vi "ThermoV_ControlSweep_NoMean_RTDCalib_160817.vi"() -> ()   [LabVIEW 2013]
panel:
  out "subarray":dbl[](array[numeric])
  out "Array":dbl[](array[numeric])
  in  "Operate HVpp\nOutput Timer":bool caption="Reset"
  out "modular 13":dbl
  in  "Number of seconds for \neach HVpp case state":dbl=30.0
  out "Elapsed Time (s)":dbl
  out "DC Value":dbl[](array[numeric]) format="%#.6f"
  in  "Saving Avg?":bool
  in  "Filename":path=path "trial_1.lvm"
  in  "STOP":bool
  out "Peak2Peak V":dbl[](array[numeric])
  out "Waveform Chart":dynamicdata(graph)
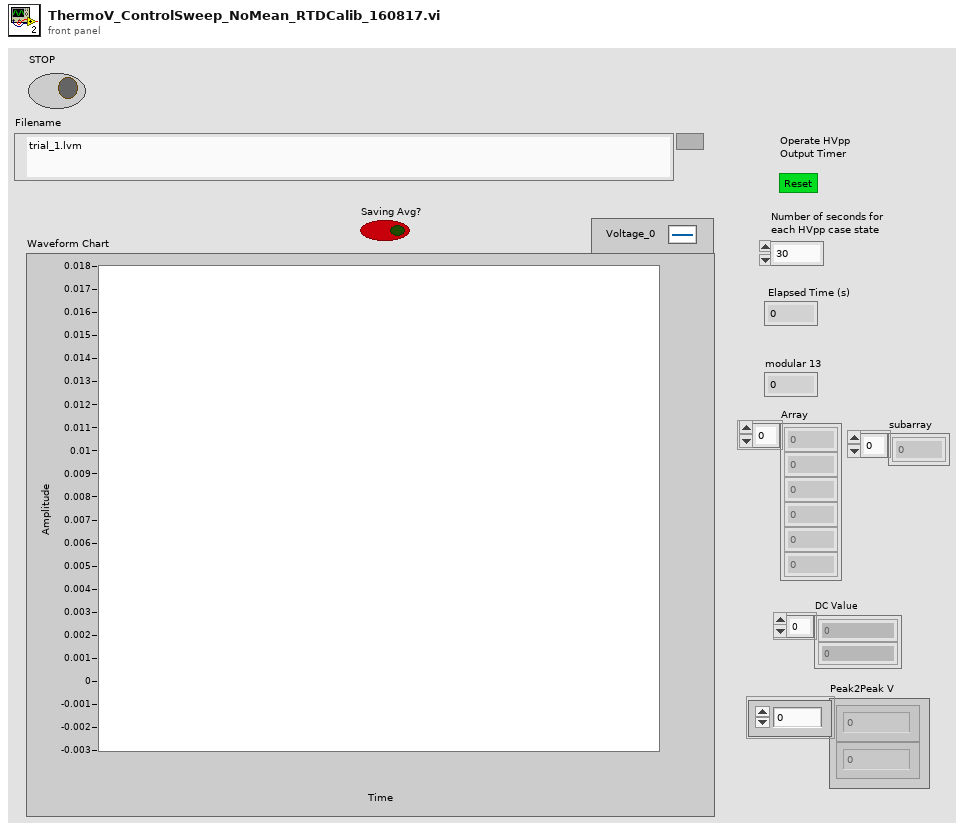
[diagram p1: front panel]
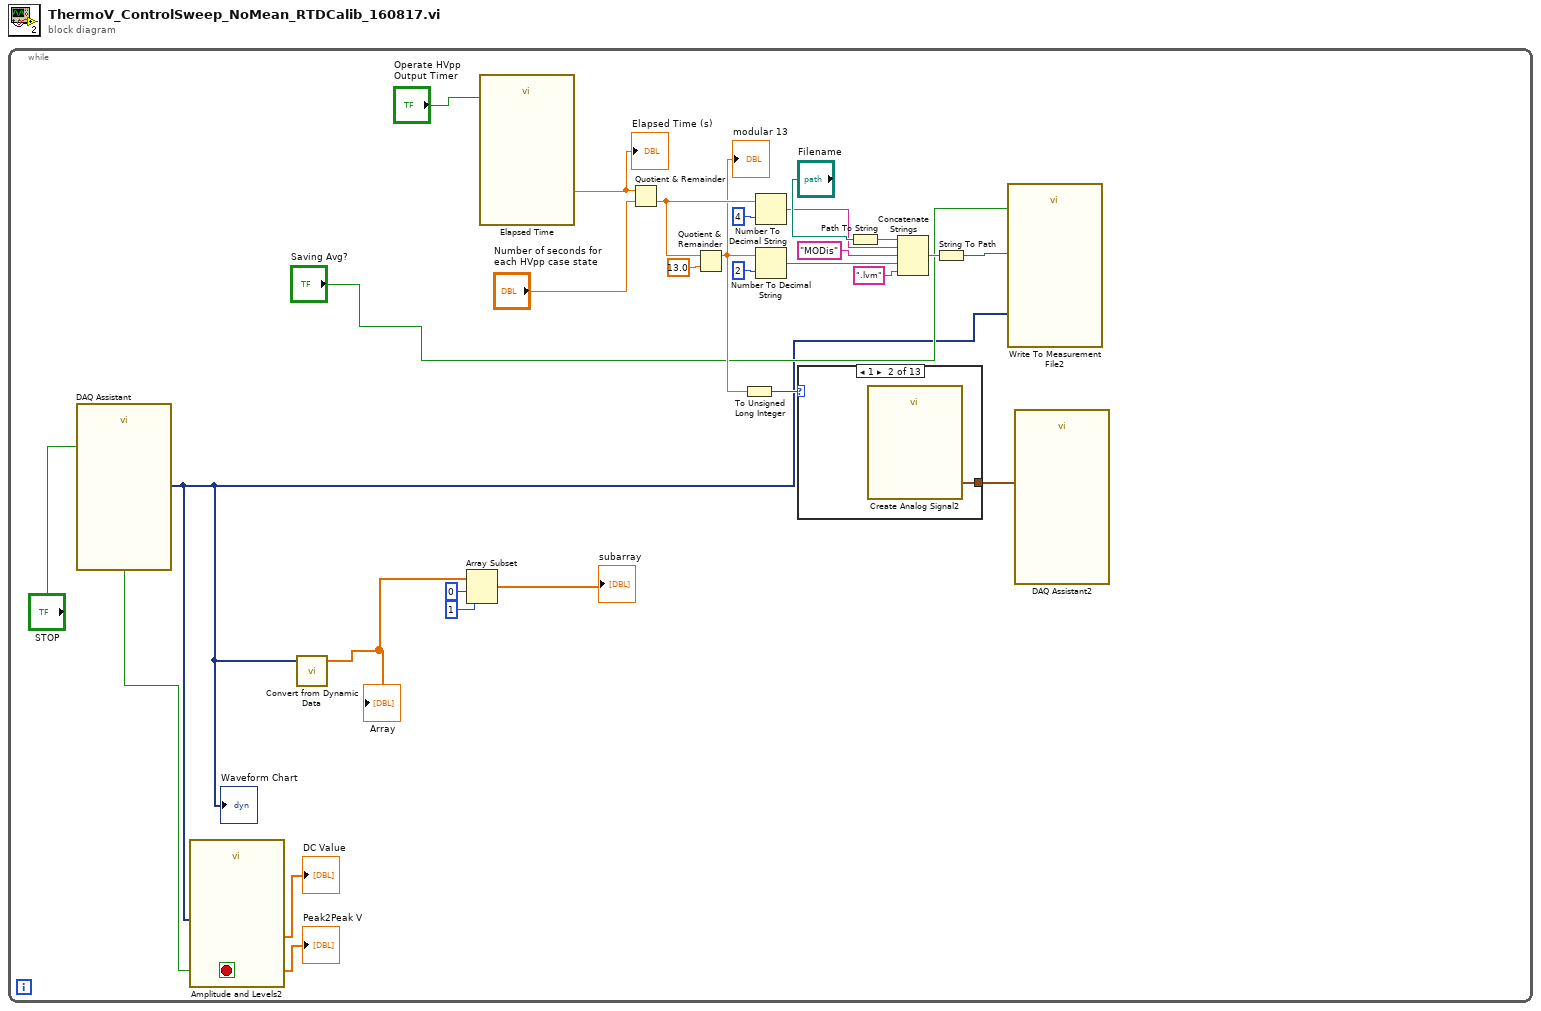
[diagram p0: block diagram]
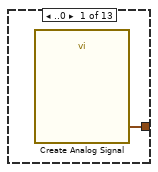
[diagram p2: hidden frame]
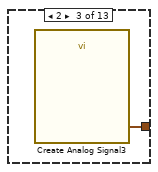
[diagram p3: hidden frame]
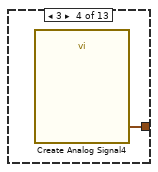
[diagram p4: hidden frame]
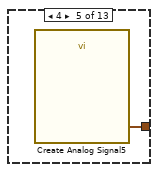
[diagram p5: hidden frame]
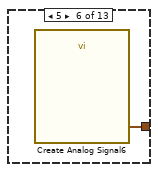
[diagram p6: hidden frame]
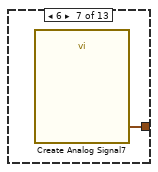
[diagram p7: hidden frame]
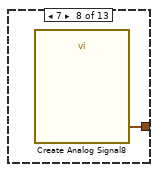
[diagram p8: hidden frame]
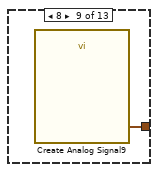
[diagram p9: hidden frame]
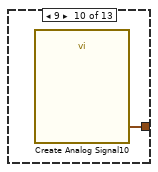
[diagram p10: hidden frame]
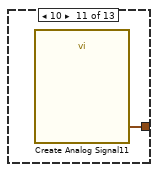
[diagram p11: hidden frame]
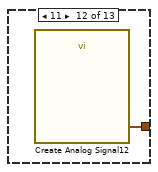
[diagram p12: hidden frame]
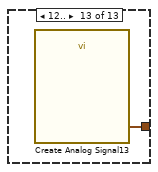
[diagram p13: hidden frame]
diagram:
  n1 = while {
    stop <- w28 stop-if-true
    n2 = call "DAQ Assistant"("stop (F)"="STOP") -> ("data"=w1:dynamicdata, "stopped"=w28:bool)  [unwired: 15 in, 2 out]
    "Waveform Chart" <- w1
    n3 = call "Amplitude and Levels2"("input signals"=w1) -> ("dc"=→"DC Value":dbl[], "peak-peak"=→"Peak2Peak V":dbl[])  [unwired: 15 in, 2 out]
    n4 = call "Convert from Dynamic Data"("Dynamic Data Type"=w1) -> ("Array"=w5:dbl[])  [unwired: 3 in]
    "Array" <- w5
    n5 = Array Subset(array=w5, index=0, length=1) -> (→"subarray":dbl[])
    n6 = call "Elapsed Time"("Reset"="Operate HVpp\nOutput Timer") -> ("Elapsed Time (s)"=w22:dbl)  [unwired: 11 in, 7 out]
    "Elapsed Time (s)" <- w22
    n7 = Quotient & Remainder(x=w22, y="Number of seconds for \neach HVpp case state") -> (floor(x/y)=w14:dbl)  [unwired: 1 out]
    n8 = Quotient & Remainder(x=w14, y=13.0) -> (x-y*floor(x/y)=w9:dbl)  [unwired: 1 out]
    "modular 13" <- w9
    n9 = To Unsigned Long Integer(number=w9) -> (unsigned 32bit integer=w23:u32)
    n10 = Number To Decimal String(number=w14, width (-)=i16 4) -> (decimal integer string=w13:string)
    n11 = Number To Decimal String(number=w9, width (-)=i16 2) -> (decimal integer string=w8:string)
    n12 = case shown="1" w23 {
      tunnel: [w29 w30 w31 w32 w33 w34 w35 w36 w37 w38 w39 w40 w41] -> w24
      frame ..0 {
        n13 = call "Create Analog Signal"() -> ("sine wave"=w29:waveform(dbl))  [unwired: 18 in, 1 out]
      }
      frame 1 {
        n14 = call "Create Analog Signal2"() -> ("sine wave"=w30:waveform(dbl))  [unwired: 18 in, 1 out]
      }
      frame 2 {
        n15 = call "Create Analog Signal3"() -> ("sine wave"=w31:waveform(dbl))  [unwired: 18 in, 1 out]
      }
      frame 3 {
        n16 = call "Create Analog Signal4"() -> ("sine wave"=w32:waveform(dbl))  [unwired: 18 in, 1 out]
      }
      frame 4 {
        n17 = call "Create Analog Signal5"() -> ("sine wave"=w33:waveform(dbl))  [unwired: 18 in, 1 out]
      }
      frame 5 {
        n18 = call "Create Analog Signal6"() -> ("sine wave"=w34:waveform(dbl))  [unwired: 18 in, 1 out]
      }
      frame 6 {
        n19 = call "Create Analog Signal7"() -> ("sine wave"=w35:waveform(dbl))  [unwired: 18 in, 1 out]
      }
      frame 7 {
        n20 = call "Create Analog Signal8"() -> ("sine wave"=w36:waveform(dbl))  [unwired: 18 in, 1 out]
      }
      frame 8 {
        n21 = call "Create Analog Signal9"() -> ("sine wave"=w37:waveform(dbl))  [unwired: 18 in, 1 out]
      }
      frame 9 {
        n22 = call "Create Analog Signal10"() -> ("sine wave"=w38:waveform(dbl))  [unwired: 18 in, 1 out]
      }
      frame 10 {
        n23 = call "Create Analog Signal11"() -> ("sine wave"=w39:waveform(dbl))  [unwired: 18 in, 1 out]
      }
      frame 11 {
        n24 = call "Create Analog Signal12"() -> ("sine wave"=w40:waveform(dbl))  [unwired: 18 in, 1 out]
      }
      frame 12.. {
        n25 = call "Create Analog Signal13"() -> ("sine wave"=w41:waveform(dbl))  [unwired: 18 in, 1 out]
      }
    }
    n26 = Path To String(path="Filename") -> (string=w16:string)
    n27 = Concatenate Strings(w16, w13, "MODis" ("string"), w8, ".lvm" ("string")) -> (w18:string)
    n28 = String To Path(string=w18) -> (path=w19:path)
    n29 = call "Write To Measurement File2"("Signals"=w1, "Enable"="Saving Avg?", "Filename"=w19) -> ()  [unwired: 14 in, 3 out]
    n30 = call "DAQ Assistant2"("data"=w24) -> ()  [unwired: 16 in, 3 out]
  }
